vi "9205_9206 16Ch Analog Input.vi"(1 "9205/6 I/O":T1={"9205/6 AI0"="NI 9205/AI0", "9205/6 AI1"="NI 9205/AI1", "9205/6 AI2"="NI 9205/AI2", "9205/6 AI3"="NI 9205/AI3", "9205/6 AI4"="NI 9205/AI4", "9205/6 AI5"="NI 9205/AI5", "9205/6 AI6"="NI 9205/AI6", "9205/6 AI7"="NI 9205/AI7", "9205/6 AI8"="NI 9205/AI8", "9205/6 AI9"="NI 9205/AI9", "9205/6 AI10"="NI 9205/AI10", "9205/6 AI11"="NI 9205/AI11", "9205/6 AI12"="NI 9205/AI12", "9205/6 AI13"="NI 9205/AI13", "9205/6 AI14"="NI 9205/AI14", "9205/6 AI15"="NI 9205/AI15"}) -> (0 "Packets":u64[](array[numeric]))   [LabVIEW 2009]
uses:
  <vilib>/eio/EIONode/EIONode.xnode
  <vilib>/rvi/eio/nirviEIOImplementation/nirviEIOImplementation.xnode
  <vilib>/rvi/eio/common/nirviEmuTemplateMethod_noerrors.vi
  <vilib>/rvi/eio/common/nirviEmuClasses.ctl
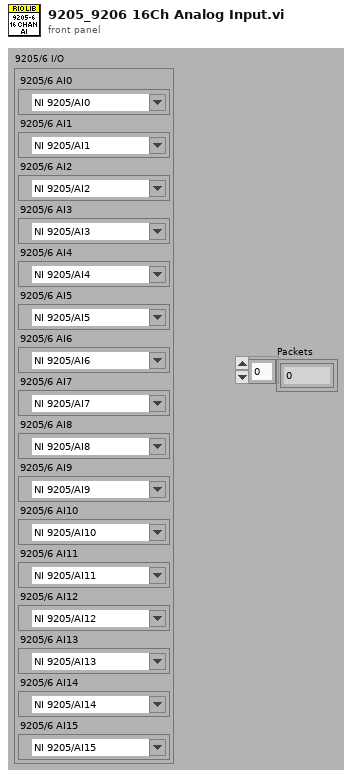
[diagram p1: front panel]
types:
  T1 = cluster{"9205/6 AI0":refnum<k21>, "9205/6 AI1":refnum<k21>, "9205/6 AI2":refnum<k21>, "9205/6 AI3":refnum<k21>, "9205/6 AI4":refnum<k21>, "9205/6 AI5":refnum<k21>, "9205/6 AI6":refnum<k21>, "9205/6 AI7":refnum<k21>, "9205/6 AI8":refnum<k21>, "9205/6 AI9":refnum<k21>, "9205/6 AI10":refnum<k21>, "9205/6 AI11":refnum<k21>, "9205/6 AI12":refnum<k21>, "9205/6 AI13":refnum<k21>, "9205/6 AI14":refnum<k21>, "9205/6 AI15":refnum<k21>}
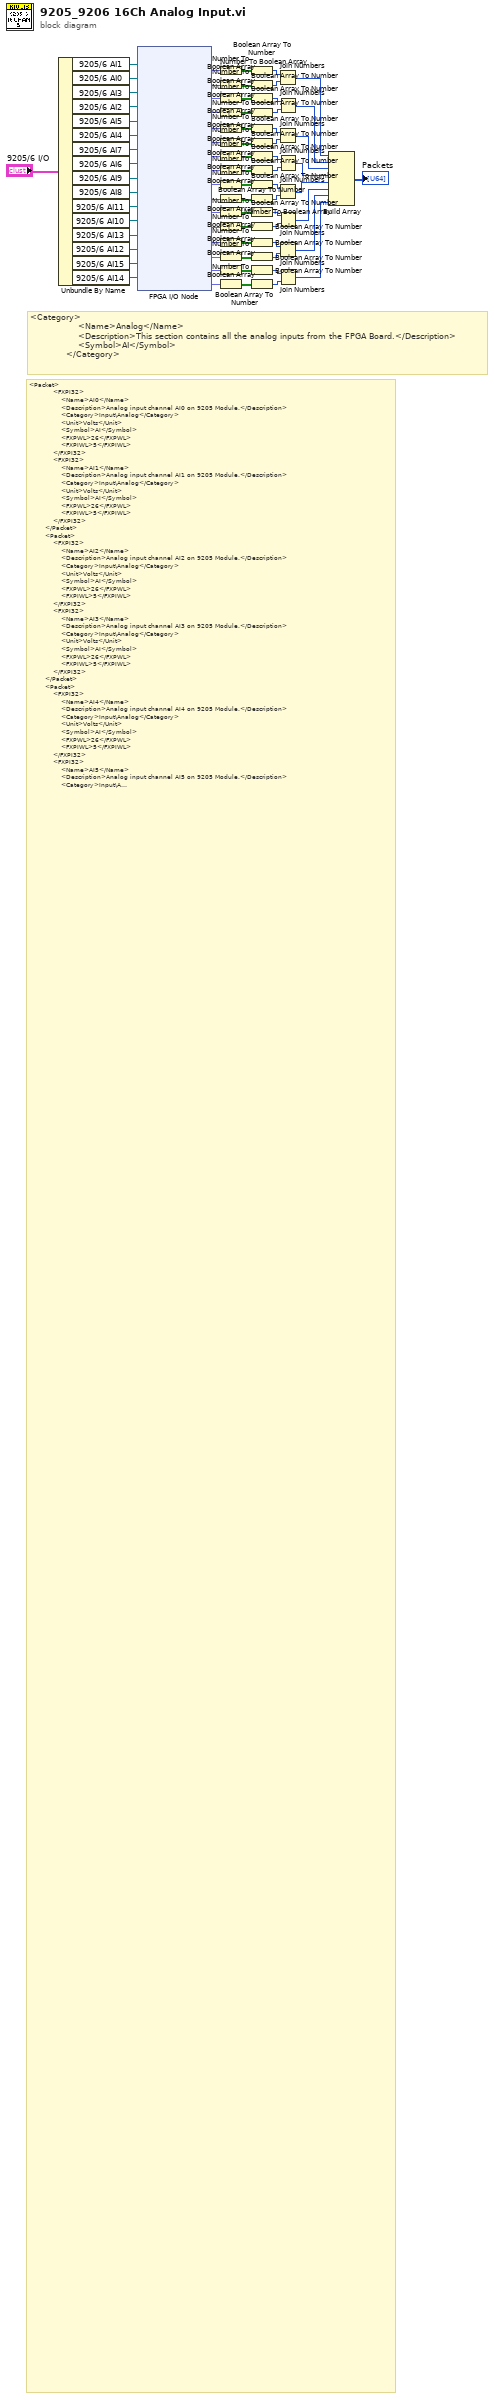
[diagram p0: block diagram]
diagram:
  # "<Category>\n                <Name>Analog</Name>\n                <Description>This section contains all the analog inputs from the FPGA Board.</Description>\n                <Symbol>AI</Symbol>\n            </Category>"
  # "<Packet>\n            <FXPI32>\n                <Name>AI0</Name>\n                <Description>Analog input channel AI0 on 9205 Module.</Description>\n                <Category>Input\\Analog</Category>\n                <Unit>Volts</Unit>\n                <Symbol>AI</Symbol>\n                <FXPWL>26</FXPWL>\n                <FXPIWL>5</FXPIWL>\n            </FXPI32>\n            <FXPI32>\n                <Name>AI1</Name>\n                <Description>Analog input channel AI1 on 9205 Module.</Description>\n                <Category>Input\\Analog</Category>\n                <Unit>Volts</Unit>\n                <Symbol>AI</Symbol>\n                <FXPWL>26</FXPWL>\n                <FXPIWL>5</FXPIWL>\n            </FXPI32>\n        </Packet>\n        <Packet>\n            <FXPI32>\n                <Name>AI2</Name>\n                <Description>Analog input channel AI2 on 9205 Module.</Description>\n                <Category>Input\\Analog</Category>\n                <Unit>Volts</Unit>\n                <Symbol>AI</Symbol>\n                <FXPWL>26</FXPWL>\n                <FXPIWL>5</FXPIWL>\n            </FXPI32>\n            <FXPI32>\n                <Name>AI3</Name>\n                <Description>Analog input channel AI3 on 9205 Module.</Description>\n                <Category>Input\\Analog</Category>\n                <Unit>Volts</Unit>\n                <Symbol>AI</Symbol>\n                <FXPWL>26</FXPWL>\n                <FXPIWL>5</FXPIWL>\n            </FXPI32>\n        </Packet>\n        <Packet>\n            <FXPI32>\n                <Name>AI4</Name>\n                <Description>Analog input channel AI4 on 9205 Module.</Description>\n                <Category>Input\\Analog</Category>\n                <Unit>Volts</Unit>\n                <Symbol>AI</Symbol>\n                <FXPWL>26</FXPWL>\n                <FXPIWL>5</FXPIWL>\n            </FXPI32>\n            <FXPI32>\n                <Name>AI5</Name>\n                <Description>Analog input channel AI5 on 9205 Module.</Description>\n                <Category>Input\\Analog</Category>\n                <Unit>Volts</Unit>\n                <Symbol>AI</Symbol>\n                <FXPWL>26</FXPWL>\n                <FXPIWL>5</FXPIWL>\n            </FXPI32>\n        </Packet>\n        <Packet>\n            <FXPI32>\n                <Name>AI6</Name>\n                <Description>Analog input channel AI6 on 9205 Module.</Description>\n                <Category>Input\\Analog</Category>\n                <Unit>Volts</Unit>\n                <Symbol>AI</Symbol>\n                <FXPWL>26</FXPWL>\n                <FXPIWL>5</FXPIWL>\n            </FXPI32>\n            <FXPI32>\n                <Name>AI7</Name>\n                <Description>Analog input channel AI7 on 9205 Module.</Description>\n                <Category>Input\\Analog</Category>\n                <Unit>Volts</Unit>\n                <Symbol>AI</Symbol>\n                <FXPWL>26</FXPWL>\n                <FXPIWL>5</FXPIWL>\n            </FXPI32>\n        </Packet>\n        <Packet>\n            <FXPI32>\n                <Name>AI8</Name>\n                <Description>Analog input channel AI8 on 9205 Module.</Description>\n                <Category>Input\\Analog</Category>\n                <Unit>Volts</Unit>\n                <Symbol>AI</Symbol>\n                <FXPWL>26</FXPWL>\n                <FXPIWL>5</FXPIWL>\n            </FXPI32>\n            <FXPI32>\n                <Name>AI9</Name>\n                <Description>Analog input channel AI9 on 9205 Module.</Description>\n                <Category>Input\\Analog</Category>\n                <Unit>Volts</Unit>\n                <Symbol>AI</Symbol>\n                <FXPWL>26</FXPWL>\n                <FXPIWL>5</FXPIWL>\n            </FXPI32>\n        </Packet>\n        <Packet>\n            <FXPI32>\n                <Name>AI10</Name>\n                <Description>Analog input channel AI10 on 9205 Module.</Description>\n                <Category>Input\\Analog</Category>\n                <Unit>Volts</Unit>\n                <Symbol>AI</Symbol>\n                <FXPWL>26</FXPWL>\n                <FXPIWL>5</FXPIWL>\n            </FXPI32>\n            <FXPI32>\n                <Name>AI11</Name>\n                <Description>Analog input channel AI11 on 9205 Module.</Description>\n                <Category>Input\\Analog</Category>\n                <Unit>Volts</Unit>\n                <Symbol>AI</Symbol>\n                <FXPWL>26</FXPWL>\n                <FXPIWL>5</FXPIWL>\n            </FXPI32>\n        </Packet>\n        <Packet>\n            <FXPI32>\n                <Name>AI12</Name>\n                <Description>Analog input channel AI12 on 9205 Module.</Description>\n                <Category>Input\\Analog</Category>\n                <Unit>Volts</Unit>\n                <Symbol>AI</Symbol>\n                <FXPWL>26</FXPWL>\n                <FXPIWL>5</FXPIWL>\n            </FXPI32>\n            <FXPI32>\n                <Name>AI13</Name>\n                <Description>Analog input channel AI13 on 9205 Module.</Description>\n                <Category>Input\\Analog</Category>\n                <Unit>Volts</Unit>\n                <Symbol>AI</Symbol>\n                <FXPWL>26</FXPWL>\n                <FXPIWL>5</FXPIWL>\n            </FXPI32>\n        </Packet>\n        <Packet>\n            <FXPI32>\n                <Name>AI14</Name>\n                <Description>Analog input channel AI14 on 9205 Module.</Description>\n                <Category>Input\\Analog</Category>\n                <Unit>Volts</Unit>\n                <Symbol>AI</Symbol>\n                <FXPWL>26</FXPWL>\n                <FXPIWL>5</FXPIWL>\n            </FXPI32>\n            <FXPI32>\n                <Name>AI15</Name>\n                <Description>Analog input channel AI15 on 9205 Module.</Description>\n                <Category>Input\\Analog</Category>\n                <Unit>Volts</Unit>\n                <Symbol>AI</Symbol>\n                <FXPWL>26</FXPWL>\n                <FXPIWL>5</FXPIWL>\n            </FXPI32>\n        </Packet>"
  n1 = Unbundle By Name("9205/6 I/O") -> ("9205/6 AI1"=w55:refnum<k21>, "9205/6 AI0"=w58:refnum<k21>, "9205/6 AI3"=w56:refnum<k21>, "9205/6 AI2"=w59:refnum<k21>, "9205/6 AI5"=w51:refnum<k21>, "9205/6 AI4"=w52:refnum<k21>, "9205/6 AI7"=w53:refnum<k21>, "9205/6 AI6"=w54:refnum<k21>, "9205/6 AI9"=w36:refnum<k21>, "9205/6 AI8"=w35:refnum<k21>, "9205/6 AI11"=w34:refnum<k21>, "9205/6 AI10"=w33:refnum<k21>, "9205/6 AI13"=w32:refnum<k21>, "9205/6 AI12"=w31:refnum<k21>, "9205/6 AI15"=w30:refnum<k21>, "9205/6 AI14"=w29:refnum<k21>)
  n2 = xnode "FPGA I/O Node"("FPGA I/O In"=w55, "FPGA I/O In"=w58, "FPGA I/O In"=w56, "FPGA I/O In"=w59, "FPGA I/O In"=w51, "FPGA I/O In"=w52, "FPGA I/O In"=w53, "FPGA I/O In"=w54, "FPGA I/O In"=w36, "FPGA I/O In"=w35, "FPGA I/O In"=w34, "FPGA I/O In"=w33, "FPGA I/O In"=w32, "FPGA I/O In"=w31, "FPGA I/O In"=w30, "FPGA I/O In"=w29) -> ("I/O Item"=w65:fxp<+/-,26,5>, "I/O Item"=w67:fxp<+/-,26,5>, "I/O Item"=w57:fxp<+/-,26,5>, "I/O Item"=w66:fxp<+/-,26,5>, "I/O Item"=w39:fxp<+/-,26,5>, "I/O Item"=w40:fxp<+/-,26,5>, "I/O Item"=w41:fxp<+/-,26,5>, "I/O Item"=w42:fxp<+/-,26,5>, "I/O Item"=w12:fxp<+/-,26,5>, "I/O Item"=w11:fxp<+/-,26,5>, "I/O Item"=w10:fxp<+/-,26,5>, "I/O Item"=w9:fxp<+/-,26,5>, "I/O Item"=w8:fxp<+/-,26,5>, "I/O Item"=w7:fxp<+/-,26,5>, "I/O Item"=w6:fxp<+/-,26,5>, "I/O Item"=w5:fxp<+/-,26,5>)  [unwired: 16 out]
  n3 = Number To Boolean Array(number=w65) -> (Boolean array=w61:bool[])
  n4 = Number To Boolean Array(number=w67) -> (Boolean array=w62:bool[])
  n5 = Number To Boolean Array(number=w57) -> (Boolean array=w64:bool[])
  n6 = Number To Boolean Array(number=w66) -> (Boolean array=w63:bool[])
  n7 = Number To Boolean Array(number=w39) -> (Boolean array=w50:bool[])
  n8 = Number To Boolean Array(number=w40) -> (Boolean array=w49:bool[])
  n9 = Number To Boolean Array(number=w41) -> (Boolean array=w47:bool[])
  n10 = Number To Boolean Array(number=w42) -> (Boolean array=w48:bool[])
  n11 = Number To Boolean Array(number=w12) -> (Boolean array=w20:bool[])
  n12 = Number To Boolean Array(number=w11) -> (Boolean array=w19:bool[])
  n13 = Number To Boolean Array(number=w10) -> (Boolean array=w17:bool[])
  n14 = Number To Boolean Array(number=w9) -> (Boolean array=w18:bool[])
  n15 = Number To Boolean Array(number=w8) -> (Boolean array=w21:bool[])
  n16 = Number To Boolean Array(number=w7) -> (Boolean array=w22:bool[])
  n17 = Number To Boolean Array(number=w6) -> (Boolean array=w24:bool[])
  n18 = Number To Boolean Array(number=w5) -> (Boolean array=w23:bool[])
  n19 = Boolean Array To Number(Boolean array=w61) -> (number=w68:u32)
  n20 = Boolean Array To Number(Boolean array=w62) -> (number=w69:u32)
  n21 = Boolean Array To Number(Boolean array=w64) -> (number=w70:u32)
  n22 = Boolean Array To Number(Boolean array=w63) -> (number=w71:u32)
  n23 = Boolean Array To Number(Boolean array=w50) -> (number=w46:u32)
  n24 = Boolean Array To Number(Boolean array=w49) -> (number=w45:u32)
  n25 = Boolean Array To Number(Boolean array=w47) -> (number=w44:u32)
  n26 = Boolean Array To Number(Boolean array=w48) -> (number=w43:u32)
  n27 = Boolean Array To Number(Boolean array=w20) -> (number=w16:u32)
  n28 = Boolean Array To Number(Boolean array=w19) -> (number=w15:u32)
  n29 = Boolean Array To Number(Boolean array=w17) -> (number=w14:u32)
  n30 = Boolean Array To Number(Boolean array=w18) -> (number=w13:u32)
  n31 = Boolean Array To Number(Boolean array=w21) -> (number=w25:u32)
  n32 = Boolean Array To Number(Boolean array=w22) -> (number=w26:u32)
  n33 = Boolean Array To Number(Boolean array=w24) -> (number=w27:u32)
  n34 = Boolean Array To Number(Boolean array=w23) -> (number=w28:u32)
  n35 = Join Numbers(hi=w68, lo=w69) -> ((hi.lo)=w72:u64)
  n36 = Join Numbers(hi=w46, lo=w45) -> ((hi.lo)=w37:u64)
  n37 = Join Numbers(hi=w16, lo=w15) -> ((hi.lo)=w1:u64)
  n38 = Join Numbers(hi=w25, lo=w26) -> ((hi.lo)=w3:u64)
  n39 = Join Numbers(hi=w70, lo=w71) -> ((hi.lo)=w73:u64)
  n40 = Join Numbers(hi=w44, lo=w43) -> ((hi.lo)=w38:u64)
  n41 = Join Numbers(hi=w14, lo=w13) -> ((hi.lo)=w2:u64)
  n42 = Join Numbers(hi=w27, lo=w28) -> ((hi.lo)=w4:u64)
  n43 = Build Array(w72, w73, w37, w38, w1, w2, w3, w4) -> (→"Packets":u64[])
